vi "Channel_low level.vi"() -> ()   [LabVIEW 2013]
uses:
  globals/Global Value.vi
panel:
  in  "VISA Refnum in":refnum<visa-resource-name>="COM3"
  in  "Channel Setting":T1(array[cluster])=[{"Channel"=1, "Gain"=4, "Shunt Resistor"=1, "Measure"=2}, {"Channel"=2, "Gain"=4, "Shunt Resistor"=5, "Measure"=1}, {"Channel"=3, "Gain"=4, "Shunt Resistor"=1, "Measure"=2}, {"Channel"=4, "Gain"=4, "Shunt Resistor"=1, "Measure"=2}, {"Channel"=6, "Gain"=4, "Shunt Resistor"=1, "Measure"=2}, {"Channel"=7, "Gain"=4, "Shunt Resistor"=5, "Measure"=1}] {"Measure" items=["Float", "Current(Diff)", "Voltage(SE+)"]; "Shunt Resistor" items=["Open"=1, "50 Ohms"=2, "500 Ohms"=3, "5k Ohms"=4, "50k Ohms"=5]; "Gain" items=["1x"=1, "10x"=2, "100x"=3, "1000x"=4]; "Channel" items=["Channel 1"=1, "Channel 2"=2, "Channel 3"=3, "Channel 4"=4, "Channel 5"=5, "Channel 6"=6, "Channel 7"=7, "Channel 8"=8]}
  # "Measure Current: Current, Shunt Resistor: 50kOhm\nMeasure Voltage: Voltage, Shunt Resistor: Open"
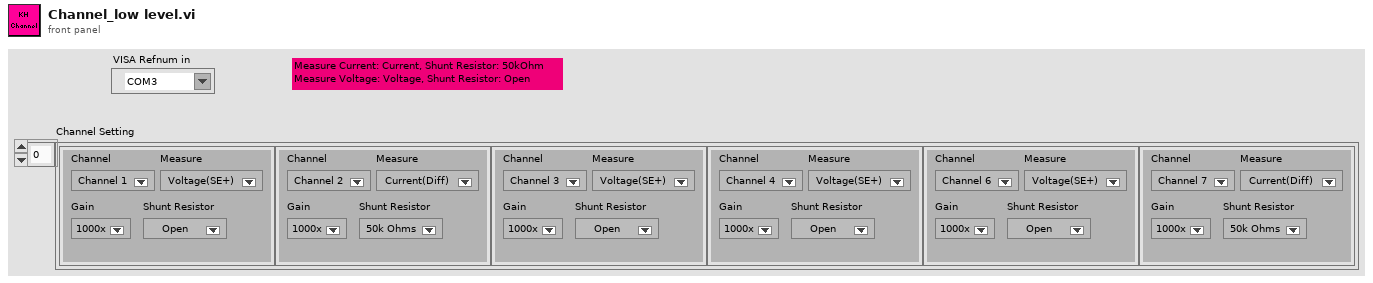
[diagram p1: front panel]
types:
  T1 = cluster{"Channel":u16, "Gain":u16, "Shunt Resistor":u16, "Measure":u16}[]
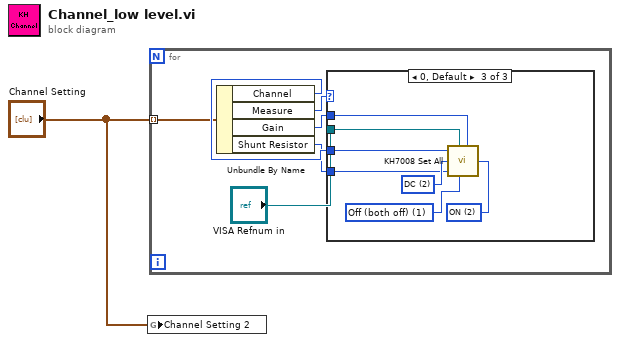
[diagram p0: block diagram]
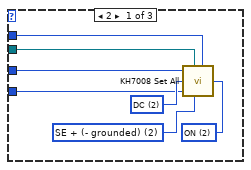
[diagram p2: hidden frame]
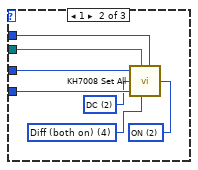
[diagram p3: hidden frame]
diagram:
  n1 = global write "Global Value.vi" "Channel Setting 2"("Channel Setting") -> ()
  n2 = for {
    tunnel: "Channel Setting" -> [w3] mode=indexing
    n3 = Unbundle By Name(w3) -> ("Channel"=w6:u16, "Measure"=w2:u16, "Gain"=w5:u16, "Shunt Resistor"=w4:u16)
    n4 = case shown="0, Default" w2 {
      tunnel: w6 -> [w11 w21 w28]
      tunnel: w5 -> [w10 w20 w27]
      tunnel: w4 -> [w9 w19 w25]
      tunnel: "VISA Refnum in" -> [w8 w15 w22]
      frame 2 {
        w12 = u16 2 items=["Off (both off)"=1, "SE + (- grounded)"=2, "SE - (+ grounded)"=3, "Diff (both on)"=4] ("Input Coupling")
        w13 = u16 2 items=["OFF"=1, "ON"=2] ("Bandwidth Filter")
        w14 = u16 2 items=["AC"=1, "DC"=2] ("Coupling")
        n5 = call "KH7008 Set All.vi"("Channel"=w11, "VISA Refnum in"=w8, "Coupling"=w14, "Shunt Resistor"=w9, "Input Coupling"=w12, "Gain"=w10, "Bandwidth Filter"=w13) -> ()  [unwired: 2 in, 1 out]
      }
      frame 1 {
        w16 = u16 2 items=["OFF"=1, "ON"=2] ("Bandwidth Filter")
        w17 = u16 4 items=["Off (both off)"=1, "SE + (- grounded)"=2, "SE - (+ grounded)"=3, "Diff (both on)"=4] ("Input Coupling")
        w18 = u16 2 items=["AC"=1, "DC"=2] ("Coupling")
        n6 = call "KH7008 Set All.vi"("Channel"=w21, "VISA Refnum in"=w15, "Coupling"=w18, "Shunt Resistor"=w19, "Input Coupling"=w17, "Gain"=w20, "Bandwidth Filter"=w16) -> ()  [unwired: 2 in, 1 out]
      }
      frame 0, Default {
        w23 = u16 2 items=["OFF"=1, "ON"=2] ("Bandwidth Filter")
        w24 = u16 1 items=["Off (both off)"=1, "SE + (- grounded)"=2, "SE - (+ grounded)"=3, "Diff (both on)"=4] ("Input Coupling")
        w26 = u16 2 items=["AC"=1, "DC"=2] ("Coupling")
        n7 = call "KH7008 Set All.vi"("Channel"=w28, "VISA Refnum in"=w22, "Coupling"=w26, "Shunt Resistor"=w25, "Input Coupling"=w24, "Gain"=w27, "Bandwidth Filter"=w23) -> ()  [unwired: 2 in, 1 out]
      }
    }
  }
